vi "handle_connection.vi"(4 "WebSocket Logger":refnum<class "WebSocket Logger.lvclass">, 6 "hangup?":refnum<notifier>, 8 "error in (no error)":errorcluster, 10 "WebSocket Connection":refnum<class "WebSocket Connection.lvclass">, 11 "WebSocket Echo Server in":refnum<class "WebSocket Echo Server.lvclass">) -> (0 "error out":errorcluster)   [LabVIEW 2019, in "WebSocket Echo Server.lvclass"]
doc: "<b>Description</b> This VI implements an \"Echo Server\" connection handler. Queries from the peer are echoed back. Additionally, the current time is sent to the peer every 10 seconds."
uses:
  WebSocket Echo Server.lvclass
  TauTerra WebSocketServer Toolkit.lvlibp/types/status_code.ctl
  TauTerra WebSocketServer Toolkit.lvlibp/classes/WebSocket Connection/WebSocket Connection.lvclass
  TauTerra WebSocketServer Toolkit.lvlibp/classes/WebSocket Logger/WebSocket Logger.lvclass
  builds/WebSocketServer Toolkit/TauTerra WebSocketServer Toolkit/TauTerra WebSocketServer Toolkit.lvlibp
panel:
  # "Handle messsages from the receive queue.\nSend messages on the send queue.\nReturn from the VI to hang-up the connection."
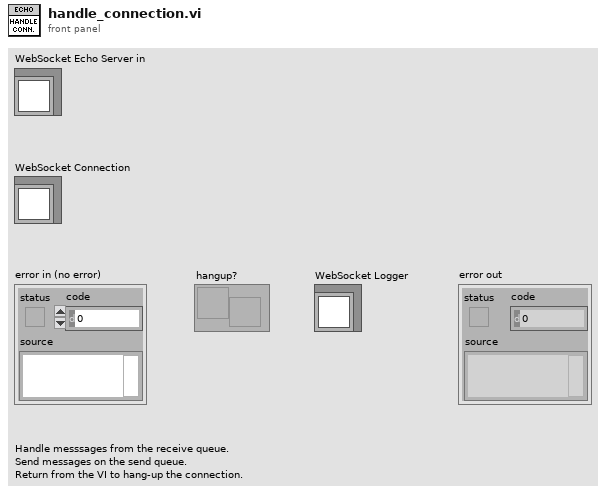
[diagram p1: front panel]
types:
  T1 = typedef "TauTerra WebSocketServer Toolkit.lvlibp/status_code.ctl" = u16
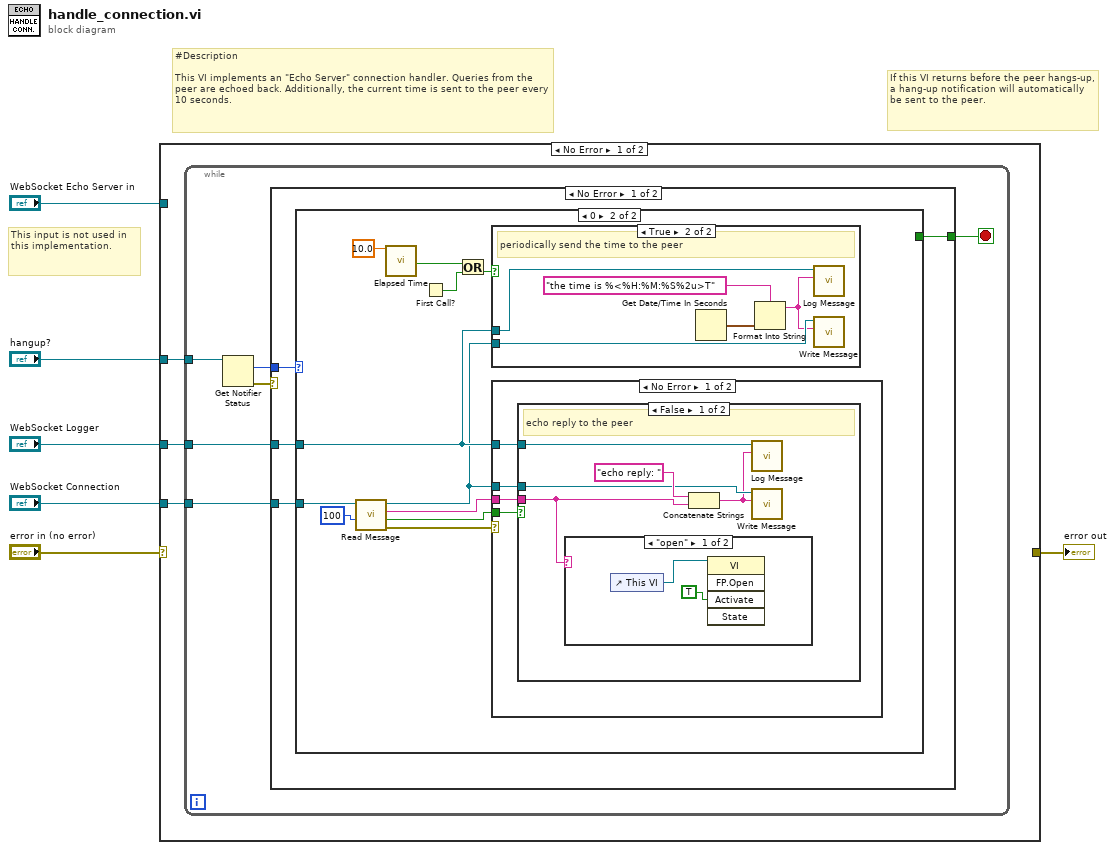
[diagram p0: block diagram]
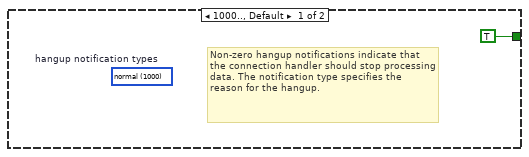
[diagram p2: hidden frame]
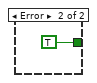
[diagram p7: hidden frame]
diagram:
  # "If this VI returns before the peer hangs-up, a hang-up notification will automatically be sent to the peer."
  # "This input is not used in this implementation."
  # "#Description\n\nThis VI implements an \"Echo Server\" connection handler. Queries from the peer are echoed back. Additionally, the current time is sent to the peer every 10 seconds."
  n1 = case shown="No Error" "error in (no error)" {
    selector: "error in (no error)" -> [_ w49]
    tunnel: [_ w49] -> w5
    tunnel: "hangup?" -> [w9 _]
    tunnel: "WebSocket Connection" -> [w8 _]
    tunnel: "WebSocket Logger" -> [w7 _]
    tunnel: "WebSocket Echo Server in" -> [_ _]
    frame No Error {
      n2 = while {
        tunnel: w9 -> [w15]
        tunnel: w8 -> [w11]
        tunnel: w7 -> [w10]
        stop <- w12 stop-if-true
        n3 = Get Notifier Status(notifier=w15) -> (current notification=w13:T1, error out=w14:errorcluster)  [unwired: 1 in, 3 out]
        n4 = case shown="No Error" w14 {
          tunnel: w13 -> [w19 _]
          tunnel: [w18 TRUE] -> w12
          tunnel: w11 -> [w17 _]
          tunnel: w10 -> [w16 _]
          frame No Error {
            n5 = case shown="0" w19 {
              tunnel: [TRUE _] -> w18
              tunnel: w17 -> [_ w31]
              tunnel: w16 -> [_ w25]
              frame 1000.., Default {
                (unwired) T1 1000 items=["ignore"=0, "normal"=1000, "going away"=1001, "protocol error"=1002, "invalid data"=1003]  # hangup notification types
                # "Non-zero hangup notifications indicate that the connection handler should stop processing data. The notification type specifies the reason for the hangup."
              }
              frame 0 {
                n6 = call "Read Message.vi"("timeout in ms (-1)"=100, "WebSocket Connection in"=w31) -> ("error out"=w28:errorcluster, "timed out?"=w27:bool, "message"=w29:string, "WebSocket Connection out"=w24:refnum<class "WebSocket Connection.lvclass">)  [unwired: 5 in, 1 out]
                n7 = call "Elapsed Time"("Time Target (s)"=10.0) -> ("Time has Elapsed"=w22:bool)  [unwired: 11 in, 7 out]
                n8 = First Call?() -> (First Call?: T/F=w21:bool)
                n9 = Or(x=w22, y=w21) -> (x .or. y?=w23:bool)
                n10 = case shown="True" w23 {
                  tunnel: w25 -> [_ w34]
                  tunnel: w24 -> [_ w33]
                  frame False {
                  }
                  frame True {
                    # "periodically send the time to the peer"
                    n11 = Get Date/Time In Seconds() -> (seconds since 1Jan1904=w35:timestamp)
                    n12 = Format Into String(format string="the time is %<%H:%M:%S%2u>T", w35) -> (resulting string=w32:string)  [unwired: 2 in, 1 out]
                    n13 = call-dynamic "Log Message.vi"("message"=w32, "WebSocket Logger in"=w34) -> ()  [unwired: 8 in, 2 out]
                    n14 = call "Write Message.vi"("message"=w32, "WebSocket Connection in"=w33) -> ()  [unwired: 8 in, 2 out]
                  }
                }
                n15 = case shown="No Error" w28 {
                  tunnel: w27 -> [w40 _]
                  tunnel: w24 -> [w39 _]
                  tunnel: w29 -> [w38 _]
                  tunnel: w25 -> [w37 _]
                  frame No Error {
                    n16 = case shown="False" w40 {
                      tunnel: w39 -> [w44 _]
                      tunnel: w38 -> [w43 _]
                      tunnel: w37 -> [w42 _]
                      frame False {
                        # "echo reply to the peer"
                        n17 = case shown="\"open\"" w43 {
                          frame "open" {
                            n18 = control-ref of="This VI"() -> (w47:refnum<vi>)
                            n19 = invoke class="VI" method="FP.Open"(reference=w47, "Activate"=TRUE ("Activate?")) -> ()  [unwired: 3 in, 5 out]
                          }
                          frame Default {
                          }
                        }
                        n20 = Concatenate Strings("echo reply: " ("string"), w43) -> (w41:string)
                        n21 = call-dynamic "Log Message.vi"("message"=w41, "WebSocket Logger in"=w42) -> ()  [unwired: 8 in, 2 out]
                        n22 = call "Write Message.vi"("message"=w41, "WebSocket Connection in"=w44) -> ()  [unwired: 8 in, 2 out]
                      }
                      frame True {
                      }
                    }
                  }
                  frame Error {
                  }
                }
              }
            }
          }
          frame Error {
          }
        }
      }
    }
    frame Error {
    }
  }
  "error out" <- w5
